vi "Remove.vi"(8 "error in":errorcluster, 11 "data sharing framework custom device":T1 format="%.0x") -> (0 "error out":errorcluster)   [LabVIEW 2019, in "Data Sharing Framework Custom Device Scripting.lvlib"]
doc: "Removes the <b>data sharing framework custom device</b> from the system definition. This removes all child threads, groups, transfer groups, transfers, and channels."
uses:
  Data Sharing Framework Custom Device Scripting.lvlib
  <vilib>/NI VeriStand/Custom Device API/Custom Device Item Ref.ctl
  NationalInstruments.VeriStand.SystemDefinitionAPI
  <vilib>/NI VeriStand/Custom Device API/Custom Device API.lvlib
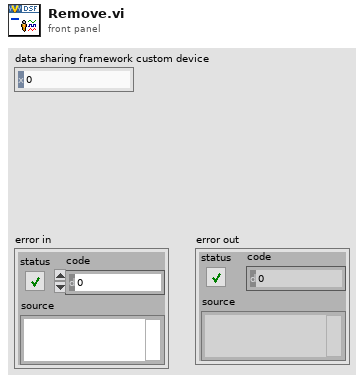
[diagram p1: front panel]
types:
  T1 = typedef "Custom Device API.lvlib/Custom Device Item Ref.ctl" = u64
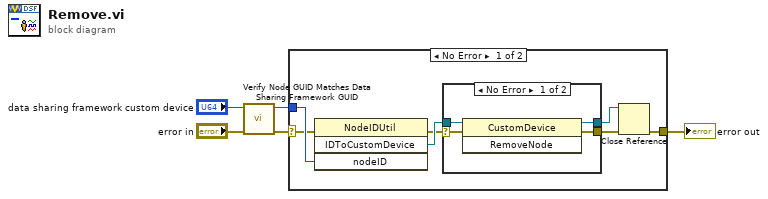
[diagram p0: block diagram]
diagram:
  n1 = call "Verify Node GUID Matches Data Sharing Framework GUID.vi"("error in"="error in", "data sharing framework custom device in"="data sharing framework custom device") -> ("error out"=w3:errorcluster, "data sharing framework custom device out"=w1:T1)  [unwired: 8 in]
  n2 = case shown="No Error" w3 {
    selector: w3 -> [w6 w19]
    tunnel: [w10 w19] -> w5
    tunnel: w1 -> [w7 _]
    frame No Error {
      n3 = invoke class="NodeIDUtil" method="IDToCustomDevice"(error in=w6, "nodeID"=w7) -> (error out=w8:errorcluster, "IDToCustomDevice"=w9:refnum<k24>)  [unwired: 2 in, 2 out]
      n4 = case shown="No Error" w8 {
        selector: w8 -> [w15 w18]
        tunnel: w9 -> [w16 w17]
        tunnel: [w14 w17] -> w12
        tunnel: [w13 w18] -> w11
        frame No Error {
          n5 = invoke class="CustomDevice" method="RemoveNode"(reference=w16, error in=w15) -> (reference out=w14:refnum<k24>, error out=w13:errorcluster)  [unwired: 1 in, 1 out]
        }
        frame Error {
        }
      }
      n6 = Close Reference(reference=w12, error in (no error)=w11) -> (error out=w10:errorcluster)
    }
    frame Error {
    }
  }
  "error out" <- w5
